vi "RLS_main.vi"(3 "dx/dt":dbl, 4 "error in (no error)":errorcluster, 5 "\\theta (t-1)":T1, 6 "u(t)":dbl, 7 "x(t)":dbl) -> (0 "error out":errorcluster, 1 "\\theta (t)":T1)   [LabVIEW 2021]
uses:
  <vilib>/Analysis/Matrix/Datatypes/RealMatrix.ctl
  <vilib>/Analysis/Matrix/NI_Matrix.lvlib
panel:
  out "x > y?":bool
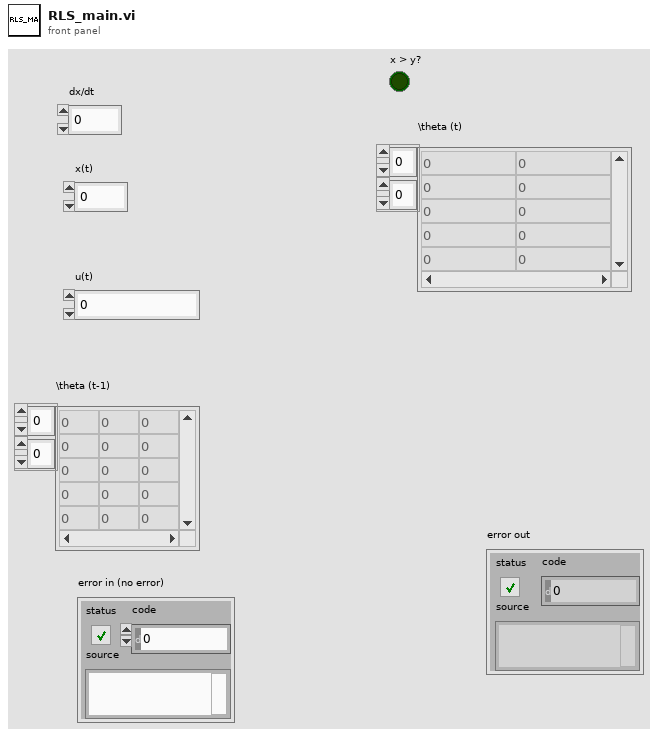
[diagram p1: front panel]
types:
  T1 = typedef "NI_Matrix.lvlib/RealMatrix.ctl" = dbl[][]
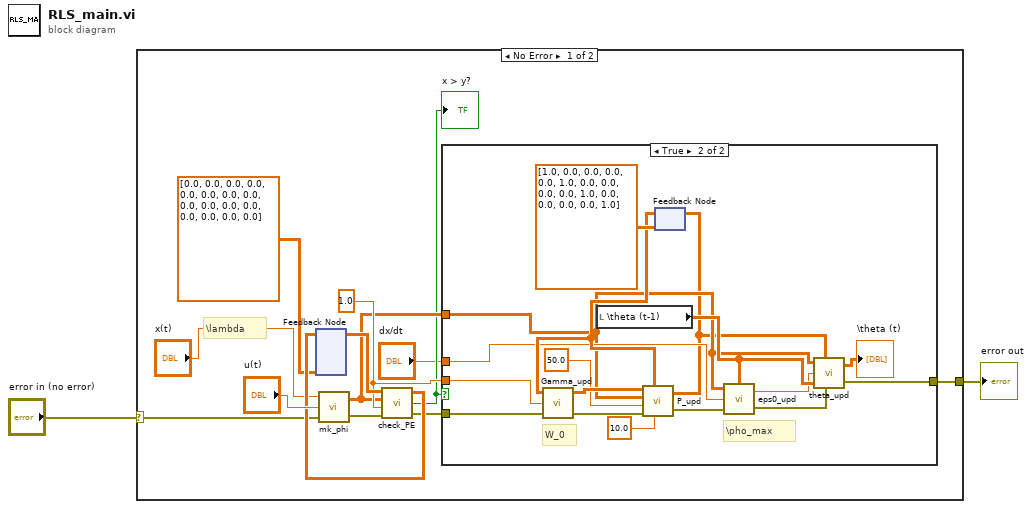
[diagram p0: block diagram]
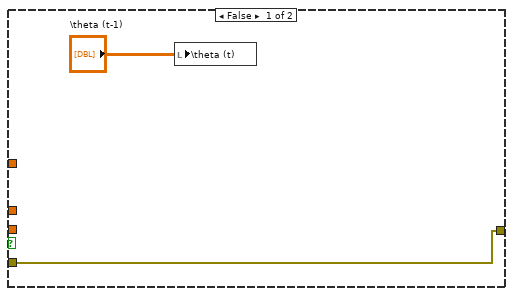
[diagram p2: hidden frame]
diagram:
  n1 = case shown="No Error" "error in (no error)" {
    selector: "error in (no error)" -> [w10 w35]
    tunnel: [w9 w35] -> w1
    frame No Error {
      w8 = 1.0 ("\\lambda")
      # "\\lambda"
      n2 = feedback #1(T1 [[0.0, 0.0, 0.0, 0.0], [0.0, 0.0, 0.0, 0.0], [0.0, 0.0, 0.0, 0.0], [0.0, 0.0, 0.0, 0.0]] ("\\Sigma (\\phi) (\\phi)^T (t)")) -> (w13:T1)
      n3 = call "mk_phi.vi"("error in (no error)"=w10, "u(t)"="u(t)", "x(t)"="x(t)") -> ("error out"=w11:errorcluster, "\\phi(t)"=w7:T1)
      n4 = call "check_PE.vi"("error in (no error)"=w11, "\\lambda"=w8, "phi(t)"=w7, "\\Sigma (phi) (phi)^T (t-1)"=w13) -> ("error out"=w3:errorcluster, "x > y?"=w6:bool, "\\Sigma (\\phi) (\\phi)^T (t)"=w14:T1)
      "x > y?" <- w6
      n5 = feedback-in #1(w14) -> ()
      n6 = case shown="True" w6 {
        tunnel: [w16 w19] -> w9
        tunnel: w3 -> [w16 w33]
        tunnel: w8 -> [_ w34]
        tunnel: w7 -> [_ w22]
        tunnel: "dx/dt" -> [_ w27]
        frame False {
          n7 = local write "\\theta (t)"("\\theta (t-1)") -> ()
        }
        frame True {
          # "\\pho_max"
          # "W_0"
          n8 = local read "\\theta (t-1)"() -> (w24:T1)
          n9 = feedback #2(T1 [[1.0, 0.0, 0.0, 0.0], [0.0, 1.0, 0.0, 0.0], [0.0, 0.0, 1.0, 0.0], [0.0, 0.0, 0.0, 1.0]] ("P(t)")) -> (w28:T1)
          n10 = call "Gamma_upd.vi"("error in (no error)"=w33, "\\lambda"=w34, "P(t-1)"=w28) -> ("error out"=w32:errorcluster, "Gamma(t)"=w30:T1)  [unwired: 1 in]
          n11 = call "P_upd.vi"("rho_max"=10.0, "P(t-1)"=w28, "error in (no error)"=w32, "W_0"=50.0, "\\phi(t)"=w22, "\\Gamma(t)"=w30) -> ("error out"=w26:errorcluster, "P(t)"=w21:T1)
          n12 = feedback-in #2(w21) -> ()
          n13 = call "eps0_upd.vi"("\\theta(t-1)"=w24, "error in (no error)"=w26, "y(t)"=w27, "\\phi(t)"=w22) -> ("error out"=w25:errorcluster, "\\eps_o(t)"=w23:dbl)
          n14 = call "theta_upd.vi"("\\phi(t)"=w22, "P(t)"=w21, "\\eps_0(t)"=w23, "\\theta(t-1)"=w24, "error in (no error)"=w25) -> ("\\theta(t)"=→"\\theta (t)":T1, "error out"=w19:errorcluster)
        }
      }
    }
    frame Error {
    }
  }
  "error out" <- w1
